vi "Create Pattern Script(BurstLength).vi"(8 "error in (no error)":errorcluster, 11 "BurstLength":T1) -> (0 "error out":errorcluster, 3 "String":string)   [LabVIEW 2018, in "BML_Frame_Root.lvclass"]
uses:
  BML_Frame_Root.lvclass
  Config_Read/BurstLength.ctl
  Config_Read/Config_Read_BML.lvclass
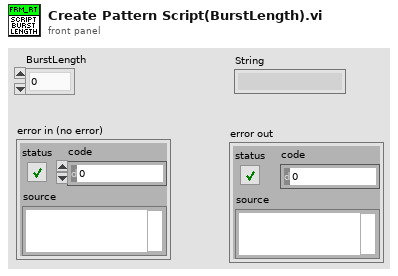
[diagram p1: front panel]
types:
  T1 = typedef "Config_Read_BML.lvclass/BurstLength.ctl" = enum8{"0", "2", "3", "4", "5", "8", "16", "32"}
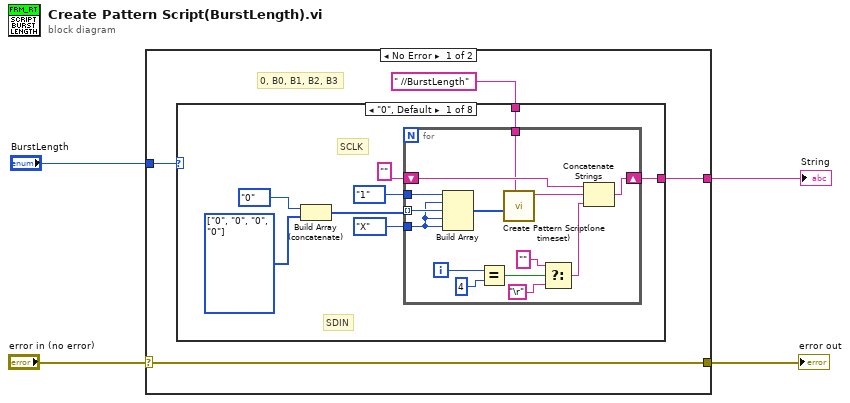
[diagram p0: block diagram]
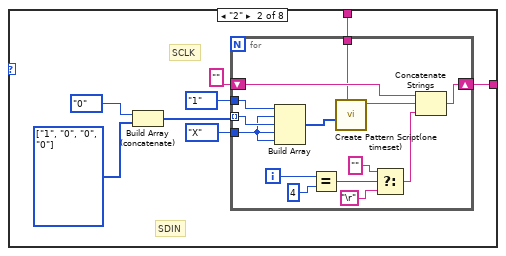
[diagram p2: hidden frame]
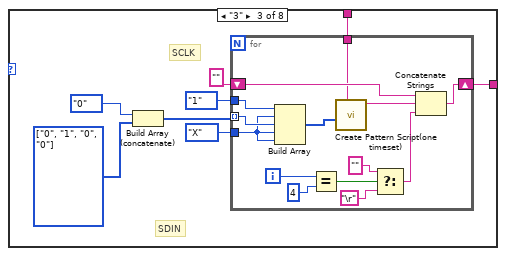
[diagram p3: hidden frame]
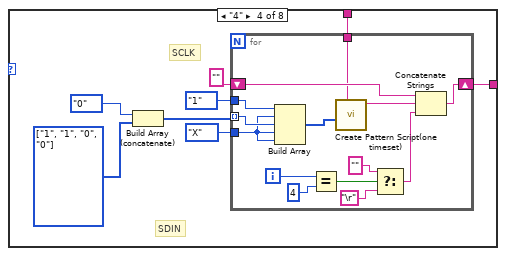
[diagram p4: hidden frame]
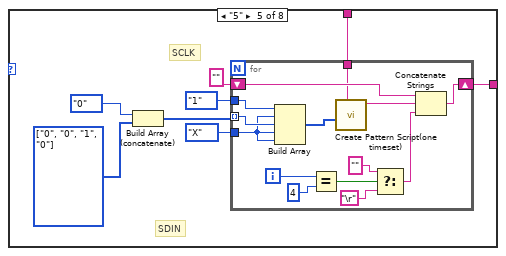
[diagram p5: hidden frame]
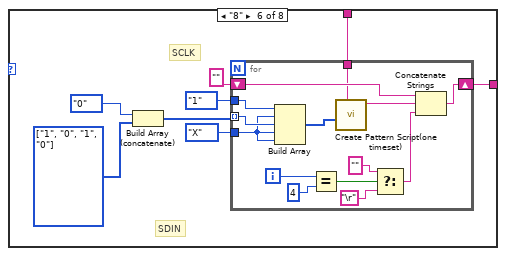
[diagram p6: hidden frame]
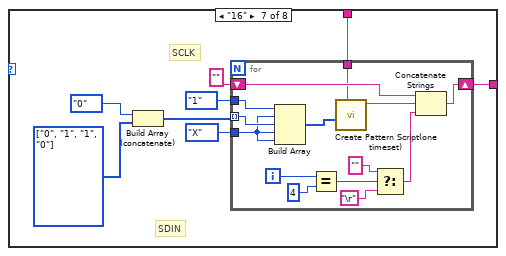
[diagram p7: hidden frame]
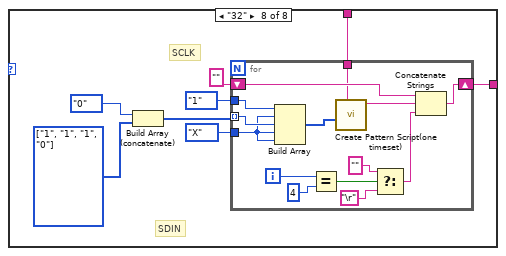
[diagram p8: hidden frame]
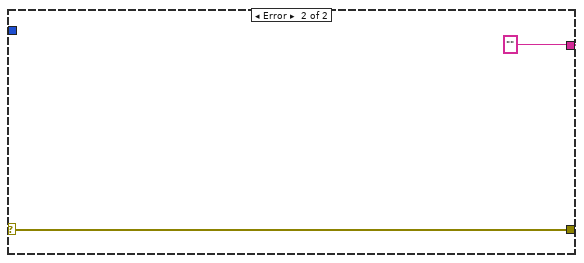
[diagram p9: hidden frame]
diagram:
  n1 = case shown="No Error" "error in (no error)" {
    selector: "error in (no error)" -> [w8 w185]
    tunnel: "BurstLength" -> [w7 _]
    tunnel: [w6 ""] -> w2
    tunnel: [w8 w185] -> w1
    frame No Error {
      # "0, B0, B1, B2, B3"
      n2 = case shown="\"0\", Default" w7 {
        tunnel: [w16 w38 w60 w82 w104 w126 w148 w170] -> w6
        tunnel: " //BurstLength" ("Notes") -> [w9 w31 w53 w75 w97 w119 w141 w163]
        frame "0", Default {
          w12 = enum16{"0", "1", "L", "H", "X", "V", "D", "M"}[] [enum."0", enum."0", enum."0", enum."0"] items=["0", "1", "L", "H", "X", "V", "D", "M"] ("PinState")
          # "SCLK"
          # "SDIN"
          n3 = Build Array (concatenate)(enum16{"0", "1", "L", "H", "X", "V", "D", "M"}."0" ("element"), w12) -> (w10:enum16{"0", "1", "L", "H", "X", "V", "D", "M"}[])
          n4 = for {
            tunnel: w10 -> [w19] mode=indexing
            shift-right: [w25] -> w16
            shift-left: "" -> [w24]
            tunnel: enum16{"0", "1", "L", "H", "X", "V", "D", "M"}."1" ("element") -> [w20]
            tunnel: enum16{"0", "1", "L", "H", "X", "V", "D", "M"}."X" ("element") -> [w18]
            tunnel: w9 -> [w17]
            i -> [w30]
            n5 = Build Array(w20, w18, w19, w18, w18) -> (w22:enum16{"0", "1", "L", "H", "X", "V", "D", "M"}[])
            n6 = Equal?(x=w30, y=4) -> (x = y?=w28:bool)
            n7 = call "Create Pattern Script(one timeset).vi"("Notes"=w17, "PinState"=w22) -> ("string out"=w21:string)  [unwired: 9 in]
            n8 = Select(t="", s=w28, f="\r") -> (s? t:f=w23:string)
            n9 = Concatenate Strings(w24, w21, w23) -> (w25:string)
          }
        }
        frame "2" {
          w32 = enum16{"0", "1", "L", "H", "X", "V", "D", "M"}[] [enum."1", enum."0", enum."0", enum."0"] items=["0", "1", "L", "H", "X", "V", "D", "M"] ("PinState")
          # "SCLK"
          # "SDIN"
          n10 = Build Array (concatenate)(enum16{"0", "1", "L", "H", "X", "V", "D", "M"}."0" ("element"), w32) -> (w33:enum16{"0", "1", "L", "H", "X", "V", "D", "M"}[])
          n11 = for {
            tunnel: w33 -> [w41] mode=indexing
            shift-right: [w47] -> w38
            shift-left: "" -> [w46]
            tunnel: enum16{"0", "1", "L", "H", "X", "V", "D", "M"}."1" ("element") -> [w42]
            tunnel: enum16{"0", "1", "L", "H", "X", "V", "D", "M"}."X" ("element") -> [w40]
            tunnel: w31 -> [w39]
            i -> [w52]
            n12 = Build Array(w42, w40, w41, w40, w40) -> (w44:enum16{"0", "1", "L", "H", "X", "V", "D", "M"}[])
            n13 = Equal?(x=w52, y=4) -> (x = y?=w50:bool)
            n14 = call "Create Pattern Script(one timeset).vi"("Notes"=w39, "PinState"=w44) -> ("string out"=w43:string)  [unwired: 9 in]
            n15 = Select(t="", s=w50, f="\r") -> (s? t:f=w45:string)
            n16 = Concatenate Strings(w46, w43, w45) -> (w47:string)
          }
        }
        frame "3" {
          w54 = enum16{"0", "1", "L", "H", "X", "V", "D", "M"}[] [enum."0", enum."1", enum."0", enum."0"] items=["0", "1", "L", "H", "X", "V", "D", "M"] ("PinState")
          # "SCLK"
          # "SDIN"
          n17 = Build Array (concatenate)(enum16{"0", "1", "L", "H", "X", "V", "D", "M"}."0" ("element"), w54) -> (w55:enum16{"0", "1", "L", "H", "X", "V", "D", "M"}[])
          n18 = for {
            tunnel: w55 -> [w63] mode=indexing
            shift-right: [w69] -> w60
            shift-left: "" -> [w68]
            tunnel: enum16{"0", "1", "L", "H", "X", "V", "D", "M"}."1" ("element") -> [w64]
            tunnel: enum16{"0", "1", "L", "H", "X", "V", "D", "M"}."X" ("element") -> [w62]
            tunnel: w53 -> [w61]
            i -> [w74]
            n19 = Build Array(w64, w62, w63, w62, w62) -> (w66:enum16{"0", "1", "L", "H", "X", "V", "D", "M"}[])
            n20 = Equal?(x=w74, y=4) -> (x = y?=w72:bool)
            n21 = call "Create Pattern Script(one timeset).vi"("Notes"=w61, "PinState"=w66) -> ("string out"=w65:string)  [unwired: 9 in]
            n22 = Select(t="", s=w72, f="\r") -> (s? t:f=w67:string)
            n23 = Concatenate Strings(w68, w65, w67) -> (w69:string)
          }
        }
        frame "4" {
          w76 = enum16{"0", "1", "L", "H", "X", "V", "D", "M"}[] [enum."1", enum."1", enum."0", enum."0"] items=["0", "1", "L", "H", "X", "V", "D", "M"] ("PinState")
          # "SCLK"
          # "SDIN"
          n24 = Build Array (concatenate)(enum16{"0", "1", "L", "H", "X", "V", "D", "M"}."0" ("element"), w76) -> (w77:enum16{"0", "1", "L", "H", "X", "V", "D", "M"}[])
          n25 = for {
            tunnel: w77 -> [w85] mode=indexing
            shift-right: [w91] -> w82
            shift-left: "" -> [w90]
            tunnel: enum16{"0", "1", "L", "H", "X", "V", "D", "M"}."1" ("element") -> [w86]
            tunnel: enum16{"0", "1", "L", "H", "X", "V", "D", "M"}."X" ("element") -> [w84]
            tunnel: w75 -> [w83]
            i -> [w96]
            n26 = Build Array(w86, w84, w85, w84, w84) -> (w88:enum16{"0", "1", "L", "H", "X", "V", "D", "M"}[])
            n27 = Equal?(x=w96, y=4) -> (x = y?=w94:bool)
            n28 = call "Create Pattern Script(one timeset).vi"("Notes"=w83, "PinState"=w88) -> ("string out"=w87:string)  [unwired: 9 in]
            n29 = Select(t="", s=w94, f="\r") -> (s? t:f=w89:string)
            n30 = Concatenate Strings(w90, w87, w89) -> (w91:string)
          }
        }
        frame "5" {
          w98 = enum16{"0", "1", "L", "H", "X", "V", "D", "M"}[] [enum."0", enum."0", enum."1", enum."0"] items=["0", "1", "L", "H", "X", "V", "D", "M"] ("PinState")
          # "SCLK"
          # "SDIN"
          n31 = Build Array (concatenate)(enum16{"0", "1", "L", "H", "X", "V", "D", "M"}."0" ("element"), w98) -> (w99:enum16{"0", "1", "L", "H", "X", "V", "D", "M"}[])
          n32 = for {
            tunnel: w99 -> [w107] mode=indexing
            shift-right: [w113] -> w104
            shift-left: "" -> [w112]
            tunnel: enum16{"0", "1", "L", "H", "X", "V", "D", "M"}."1" ("element") -> [w108]
            tunnel: enum16{"0", "1", "L", "H", "X", "V", "D", "M"}."X" ("element") -> [w106]
            tunnel: w97 -> [w105]
            i -> [w118]
            n33 = Build Array(w108, w106, w107, w106, w106) -> (w110:enum16{"0", "1", "L", "H", "X", "V", "D", "M"}[])
            n34 = Equal?(x=w118, y=4) -> (x = y?=w116:bool)
            n35 = call "Create Pattern Script(one timeset).vi"("Notes"=w105, "PinState"=w110) -> ("string out"=w109:string)  [unwired: 9 in]
            n36 = Select(t="", s=w116, f="\r") -> (s? t:f=w111:string)
            n37 = Concatenate Strings(w112, w109, w111) -> (w113:string)
          }
        }
        frame "8" {
          w120 = enum16{"0", "1", "L", "H", "X", "V", "D", "M"}[] [enum."1", enum."0", enum."1", enum."0"] items=["0", "1", "L", "H", "X", "V", "D", "M"] ("PinState")
          # "SCLK"
          # "SDIN"
          n38 = Build Array (concatenate)(enum16{"0", "1", "L", "H", "X", "V", "D", "M"}."0" ("element"), w120) -> (w121:enum16{"0", "1", "L", "H", "X", "V", "D", "M"}[])
          n39 = for {
            tunnel: w121 -> [w129] mode=indexing
            shift-right: [w135] -> w126
            shift-left: "" -> [w134]
            tunnel: enum16{"0", "1", "L", "H", "X", "V", "D", "M"}."1" ("element") -> [w130]
            tunnel: enum16{"0", "1", "L", "H", "X", "V", "D", "M"}."X" ("element") -> [w128]
            tunnel: w119 -> [w127]
            i -> [w140]
            n40 = Build Array(w130, w128, w129, w128, w128) -> (w132:enum16{"0", "1", "L", "H", "X", "V", "D", "M"}[])
            n41 = Equal?(x=w140, y=4) -> (x = y?=w138:bool)
            n42 = call "Create Pattern Script(one timeset).vi"("Notes"=w127, "PinState"=w132) -> ("string out"=w131:string)  [unwired: 9 in]
            n43 = Select(t="", s=w138, f="\r") -> (s? t:f=w133:string)
            n44 = Concatenate Strings(w134, w131, w133) -> (w135:string)
          }
        }
        frame "16" {
          w142 = enum16{"0", "1", "L", "H", "X", "V", "D", "M"}[] [enum."0", enum."1", enum."1", enum."0"] items=["0", "1", "L", "H", "X", "V", "D", "M"] ("PinState")
          # "SCLK"
          # "SDIN"
          n45 = Build Array (concatenate)(enum16{"0", "1", "L", "H", "X", "V", "D", "M"}."0" ("element"), w142) -> (w143:enum16{"0", "1", "L", "H", "X", "V", "D", "M"}[])
          n46 = for {
            tunnel: w143 -> [w151] mode=indexing
            shift-right: [w157] -> w148
            shift-left: "" -> [w156]
            tunnel: enum16{"0", "1", "L", "H", "X", "V", "D", "M"}."1" ("element") -> [w152]
            tunnel: enum16{"0", "1", "L", "H", "X", "V", "D", "M"}."X" ("element") -> [w150]
            tunnel: w141 -> [w149]
            i -> [w162]
            n47 = Build Array(w152, w150, w151, w150, w150) -> (w154:enum16{"0", "1", "L", "H", "X", "V", "D", "M"}[])
            n48 = Equal?(x=w162, y=4) -> (x = y?=w160:bool)
            n49 = call "Create Pattern Script(one timeset).vi"("Notes"=w149, "PinState"=w154) -> ("string out"=w153:string)  [unwired: 9 in]
            n50 = Select(t="", s=w160, f="\r") -> (s? t:f=w155:string)
            n51 = Concatenate Strings(w156, w153, w155) -> (w157:string)
          }
        }
        frame "32" {
          w164 = enum16{"0", "1", "L", "H", "X", "V", "D", "M"}[] [enum."1", enum."1", enum."1", enum."0"] items=["0", "1", "L", "H", "X", "V", "D", "M"] ("PinState")
          # "SCLK"
          # "SDIN"
          n52 = Build Array (concatenate)(enum16{"0", "1", "L", "H", "X", "V", "D", "M"}."0" ("element"), w164) -> (w165:enum16{"0", "1", "L", "H", "X", "V", "D", "M"}[])
          n53 = for {
            tunnel: w165 -> [w173] mode=indexing
            shift-right: [w179] -> w170
            shift-left: "" -> [w178]
            tunnel: enum16{"0", "1", "L", "H", "X", "V", "D", "M"}."1" ("element") -> [w174]
            tunnel: enum16{"0", "1", "L", "H", "X", "V", "D", "M"}."X" ("element") -> [w172]
            tunnel: w163 -> [w171]
            i -> [w184]
            n54 = Build Array(w174, w172, w173, w172, w172) -> (w176:enum16{"0", "1", "L", "H", "X", "V", "D", "M"}[])
            n55 = Equal?(x=w184, y=4) -> (x = y?=w182:bool)
            n56 = call "Create Pattern Script(one timeset).vi"("Notes"=w171, "PinState"=w176) -> ("string out"=w175:string)  [unwired: 9 in]
            n57 = Select(t="", s=w182, f="\r") -> (s? t:f=w177:string)
            n58 = Concatenate Strings(w178, w175, w177) -> (w179:string)
          }
        }
      }
    }
    frame Error {
    }
  }
  "String" <- w2
  "error out" <- w1
